vi "Update Data's to Ctrl & Indicator's.vi"(7 "Data Cluster In":T1, 8 "error in (no error)":errorcluster) -> (0 "error out":errorcluster, 5 "Data Cluster Out":T1)   [LabVIEW 2021, in "Test Panel GUI Update.lvlib"]
doc: "<b>Note:</b> This VI was modified by the <b>Validate DQMH Module</b> tool to turn off automatic error handling."
uses:
  Test Panel GUI Update.lvlib
  Module Data--cluster.ctl
  Test Panel/GUI Ctrl Data's--Cluster.ctl
  Test Panel/Rx-Mapping Data.ctl
  Capsule-Data's.ctl
  Host-Control's/DIO Data's from RT.ctl
  Host-Control's/AI-Data from RT.ctl
  Test Panel/Test Panel.lvlib
panel:
  out "Array 2":bool[](array[boolean])
  out "Array":errorcluster[](array[cluster])
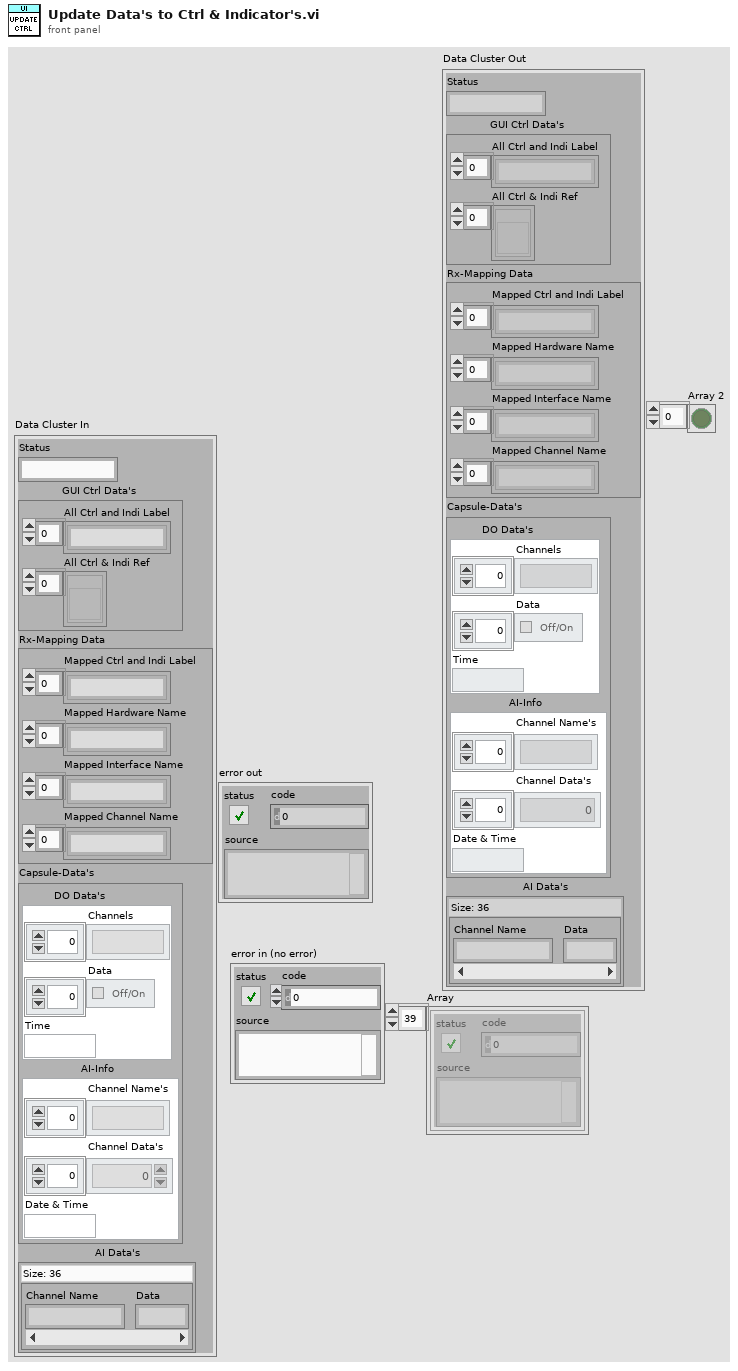
[diagram p1: front panel]
types:
  T1 = typedef "Test Panel GUI Update.lvlib/Module Data--cluster.ctl" = cluster{"Status":string, "GUI Ctrl Data's":T2, "Rx-Mapping Data":T3, "Capsule-Data's":T4, "AI Data's":map{string, dbl}}
  T2 = typedef "Test Panel.lvlib/GUI Ctrl Data's--Cluster.ctl" = cluster{"All Ctrl and Indi Label":string[], "All Ctrl & Indi Ref":refnum<vi>[]}
  T3 = typedef "Test Panel.lvlib/Rx-Mapping Data.ctl" = cluster{"Mapped Ctrl and Indi Label":string[], "Mapped Hardware Name":string[], "Mapped Interface Name":string[], "Mapped Channel Name":string[]}
  T4 = typedef "Test Panel GUI Update.lvlib/Capsule-Data's.ctl" = cluster{"DIO Data's":T5, "AI-Info":T6}
  T5 = typedef "DIO Data's from RT.ctl" = cluster{"Channels":string[], "Data":bool[], "Time":string}
  T6 = typedef "AI-Data from RT.ctl" = cluster{"Channel Name's":string[], "Channel Data's":dbl[], "Date & Time":string}
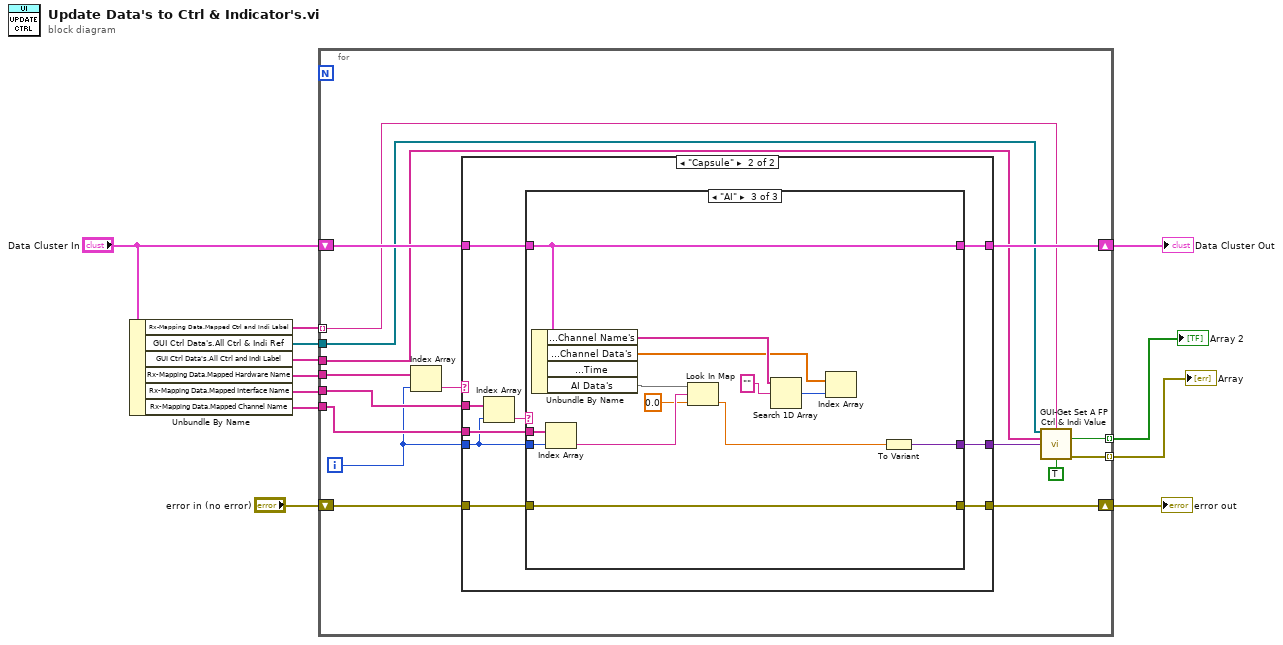
[diagram p0: block diagram]
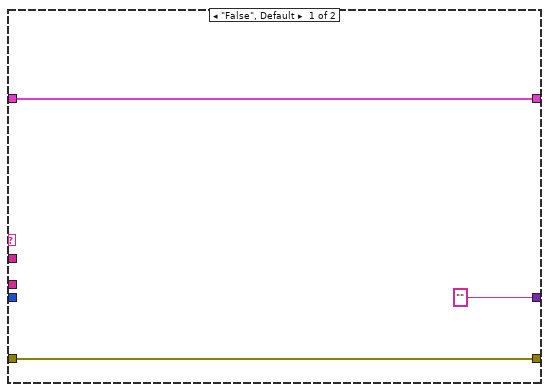
[diagram p2: hidden frame]
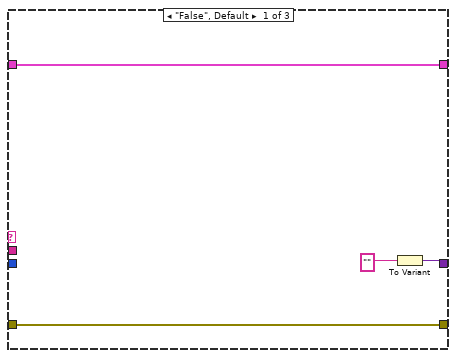
[diagram p3: hidden frame]
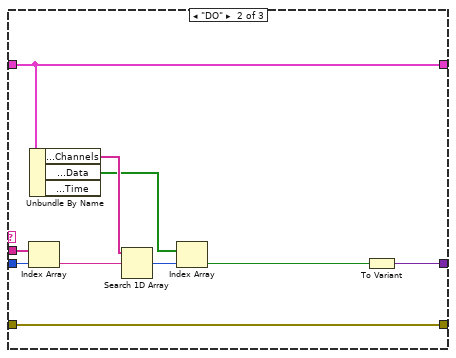
[diagram p4: hidden frame]
diagram:
  n1 = Unbundle By Name("Data Cluster In") -> ("Rx-Mapping Data.Mapped Ctrl and Indi Label"=w3:string[], "GUI Ctrl Data's.All Ctrl & Indi Ref"=w4:refnum<vi>[], "GUI Ctrl Data's.All Ctrl and Indi Label"=w9:string[], "Rx-Mapping Data.Mapped Hardware Name"=w10:string[], "Rx-Mapping Data.Mapped Interface Name"=w12:string[], "Rx-Mapping Data.Mapped Channel Name"=w11:string[])
  n2 = for {
    tunnel: w9 -> [w20]
    tunnel: w3 -> [w19] mode=indexing
    tunnel: w12 -> [w27]
    tunnel: w11 -> [w26]
    tunnel: w10 -> [w28]
    shift-right: [w15] -> w7
    shift-left: "error in (no error)" -> [w25]
    shift-right: [w23] -> w5
    shift-left: "Data Cluster In" -> [w24]
    tunnel: w4 -> [w21]
    tunnel: [w14] -> w2 mode=indexing
    tunnel: [w13] -> w1 mode=indexing
    i -> [w22]
    n3 = Index Array(array=w28, index=w22) -> (element=w18:string)
    n4 = case shown="\"Capsule\"" w18 {
      tunnel: w27 -> [_ w40]
      tunnel: w22 -> [_ w33]
      tunnel: w26 -> [_ w38]
      tunnel: w25 -> [w31 w37]
      tunnel: [w31 w36] -> w15
      tunnel: ["" ("Label.Text") w32] -> w17
      tunnel: w24 -> [w29 w35]
      tunnel: [w29 w34] -> w23
      frame "False", Default {
      }
      frame "Capsule" {
        n5 = Index Array(array=w40, index=w33) -> (element=w39:string)
        n6 = case shown="\"AI\"" w39 {
          tunnel: w38 -> [_ w54 w67]
          tunnel: w33 -> [_ w53 w66]
          tunnel: w37 -> [w44 w50 w64]
          tunnel: [w44 w50 w64] -> w36
          tunnel: w35 -> [w43 w49 w63]
          tunnel: [w43 w49 w63] -> w34
          tunnel: [w41 w46 w60] -> w32
          frame "False", Default {
            n7 = To Variant(anything="" ("Label.Text")) -> (Variant=w41:variant)
          }
          frame "DO" {
            n8 = Index Array(array=w54, index=w53) -> (element=w52:string)
            n9 = Unbundle By Name(w49) -> ("Capsule-Data's.DIO Data's.Channels"=w48:string[], "Capsule-Data's.DIO Data's.Data"=w47:bool[])  [unwired: 1 out]
            n10 = Search 1D Array(1D array=w48, element=w52) -> (index of element=w51:i32)  [unwired: 1 in]
            n11 = Index Array(array=w47, index=w51) -> (element=w45:bool)
            n12 = To Variant(anything=w45) -> (Variant=w46:variant)
          }
          frame "AI" {
            n13 = Unbundle By Name(w63) -> ("Capsule-Data's.AI-Info.Channel Name's"=w62:string[], "Capsule-Data's.AI-Info.Channel Data's"=w61:dbl[], "AI Data's"=w59:map{string, dbl})  [unwired: 1 out]
            n14 = Index Array(array=w67, index=w66) -> (element=w58:string)
            n15 = Look In Map(map=w59, key=w58, default value=0.0) -> (value=w56:dbl)  [unwired: 1 out]
            n16 = Search 1D Array(1D array=w62, element="") -> (index of element=w65:i32)  [unwired: 1 in]
            n17 = Index Array(array=w61, index=w65) -> ()  [unwired: 1 out]
            n18 = To Variant(anything=w56) -> (Variant=w60:variant)
          }
        }
      }
    }
    n19 = call "GUI-Get Set A FP Ctrl & Indi Value.vi"("All Object Ref"=w21, "Label"=w19, "All Object Label"=w20, "Ctrl Value In"=w17, "Set(F)"=TRUE) -> ("Refnum OK?"=w13:bool, "error out"=w14:errorcluster)  [unwired: 7 in, 2 out]
  }
  "error out" <- w7
  "Data Cluster Out" <- w5
  "Array" <- w2
  "Array 2" <- w1
